vi "Annotation VLine.vi"(4 "label":string, 9 "Marker Options":T1={"Color"=16723218, "Text"="Drag and click to position a marker", "Type"=enum."point", "pen"={"Width"=2, "Style"=enum."Solid"}, "font"={"Font Name"="Arial", "Size"=16, "Strikeout?"=FALSE, "Italic?"=FALSE, "Underline?"=FALSE, "Outline?"=FALSE, "Shadow?"=FALSE, "Bold?"=FALSE, "Color Box"=0}}, 10 "position":T2, 11 "picture":picture) -> (3 "new picture":picture)   [LabVIEW 2015]
doc: "Draw the verticle line for showing notes"
uses:
  <vilib>/Utility/miscctls.llb/LVPoint32TypeDef.ctl
  controls/AnnotationOptions.ctl
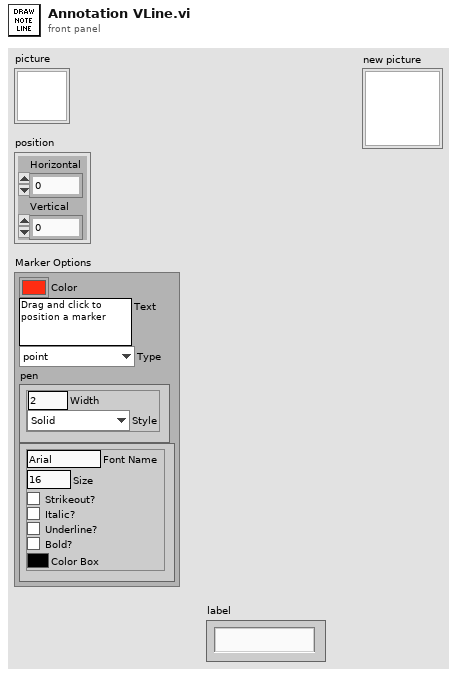
[diagram p1: front panel]
types:
  T1 = typedef "AnnotationOptions.ctl" = cluster{"Color":u32, "Text":string, "Type":enum16{"point", "horiz", "vert", "vert range", "horiz range", "box"}, "pen":cluster{"Width":u16, "Style":enum32{"Solid", "Dash", "Dot", "DashDot", "DashDotDot"}}, "font":cluster{"Font Name":string, "Size":i16, "Strikeout?":bool, "Italic?":bool, "Underline?":bool, "Outline?":bool, "Shadow?":bool, "Bold?":bool, "Color Box":u32}}
  T2 = typedef "LVPoint32TypeDef.ctl" = cluster{"Horizontal":i32, "Vertical":i32}
  T3 = cluster{"Font Name:":string, "Size":i16, "Strikeout?":bool, "Italic?":bool, "Underline?":bool, "Outline?":bool, "Shadow?":bool, "Bold?":bool}
  T4 = enum16{"User-specified Font", "Application Font", "System Font", "Dialog Font"}
  T5 = cluster{"Width":u16, "Style":enum32{"Solid", "Dash", "Dot", "DashDot", "DashDotDot"}}
  T6 = cluster{"Font Name":string, "Size":i16, "Strikeout?":bool, "Italic?":bool, "Underline?":bool, "Outline?":bool, "Shadow?":bool, "Bold?":bool, "Color Box":u32}
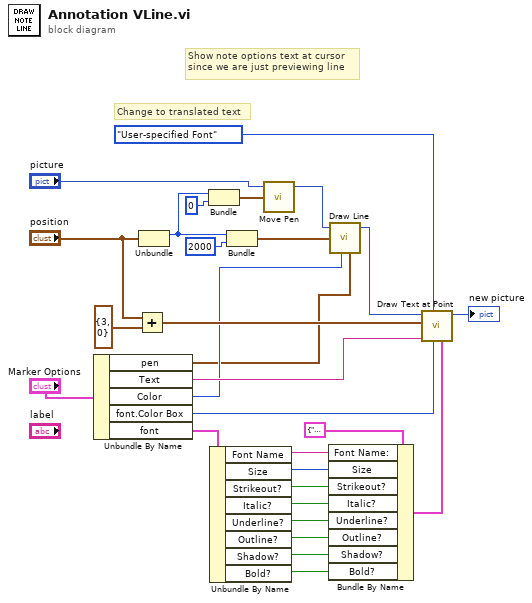
[diagram p0: block diagram]
diagram:
  # "Show note options text at cursor\nsince we are just previewing line"
  # "Change to translated text"
  n1 = Unbundle By Name("Marker Options") -> ("pen"=w1:T5, "Text"=w15:string, "Color"=w14:u32, "font.Color Box"=w13:u32, "font"=w12:T6)
  n2 = Add(x="position", y=T2 {"Horizontal"=3, "Vertical"=0}) -> (x+y=w27:T2)
  n3 = Unbundle("position") -> ("Horizontal"=w26:i32)  [unwired: 1 out]
  n4 = Bundle("Horizontal"=w26, "top"=i16 0) -> (w19:cluster{"Horizontal":i32, "top":i16})  [unwired: 1 in]
  n5 = Unbundle By Name(w12) -> ("Font Name"=w10:string, "Size"=w9:i16, "Strikeout?"=w8:bool, "Italic?"=w7:bool, "Underline?"=w6:bool, "Outline?"=w5:bool, "Shadow?"=w4:bool, "Bold?"=w3:bool)
  n6 = Bundle("Horizontal"=w26, "top"=i16 2000) -> (w25:cluster{"Horizontal":i32, "top":i16})  [unwired: 1 in]
  n7 = call <vilib>:"Move Pen.vi"("new position"=w19, "picture"="picture") -> ("new picture"=w22:picture)  [unwired: 3 in]
  n8 = Bundle By Name(cluster=T3 {"Font Name:"="", "Size"=12, "Strikeout?"=FALSE, "Italic?"=FALSE, "Underline?"=FALSE, "Outline?"=FALSE, "Shadow?"=FALSE, "Bold?"=FALSE} ("[user-specified font]"), "Font Name:"=w10, "Size"=w9, "Strikeout?"=w8, "Italic?"=w7, "Underline?"=w6, "Outline?"=w5, "Shadow?"=w4, "Bold?"=w3) -> (w2:T3)
  n9 = call <vilib>:"Draw Line.vi"("picture"=w22, "end point"=w25, "color(black)"=w14, "pen"=w1) -> ("new picture"=w23:picture)  [unwired: 5 in]
  n10 = call <vilib>:"Draw Text at Point.vi"("[user-specified font]"=w2, "text color(black)"=w13, "desired font(Application)"=T4."User-specified Font", "text"=w15, "origin"=w27, "picture"=w23) -> ("new picture"=→"new picture":picture)  [unwired: 4 in, 1 out]
